vi "Modified Traverse Positions.vi"(4 "Input Position":sgl[](array[numeric])=[0.0, 0.0, 0.0] format="%.2f", 5 "Simulate/Run":T1, 6 "Work in Tunnel Coordinates?":T2, 7 "Extra Command String":string) -> (0 "Error String":string, 1 "XYZ Offset of 2nd Traverse":sgl[](array[numeric]), 2 "Traverse Positions":sgl[][](array[numeric]) format="%.2f", 3 "Traverse Setups":string[](array[string]))   [LabVIEW 2018]
uses:
  Controls/Tunnel_Coordinates.ctl
  Controls/User_Specific_mode.ctl
  Globals/Trav_pos_global.vi
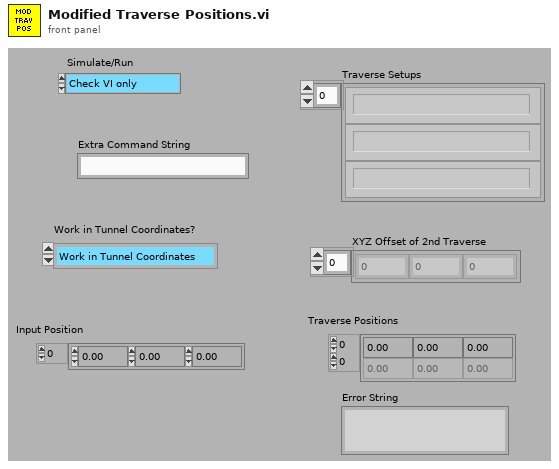
[diagram p1: front panel]
types:
  T1 = typedef "User_Specific_mode.ctl" = enum16{"Check VI only", "Run VI"}
  T2 = typedef "Tunnel_Coordinates.ctl" = enum16{"Work in Tunnel Coordinates", "Work in Model Coordinates"}
  T3 = enum16{"To Traverse Coordinates", "To User Coordinates"}
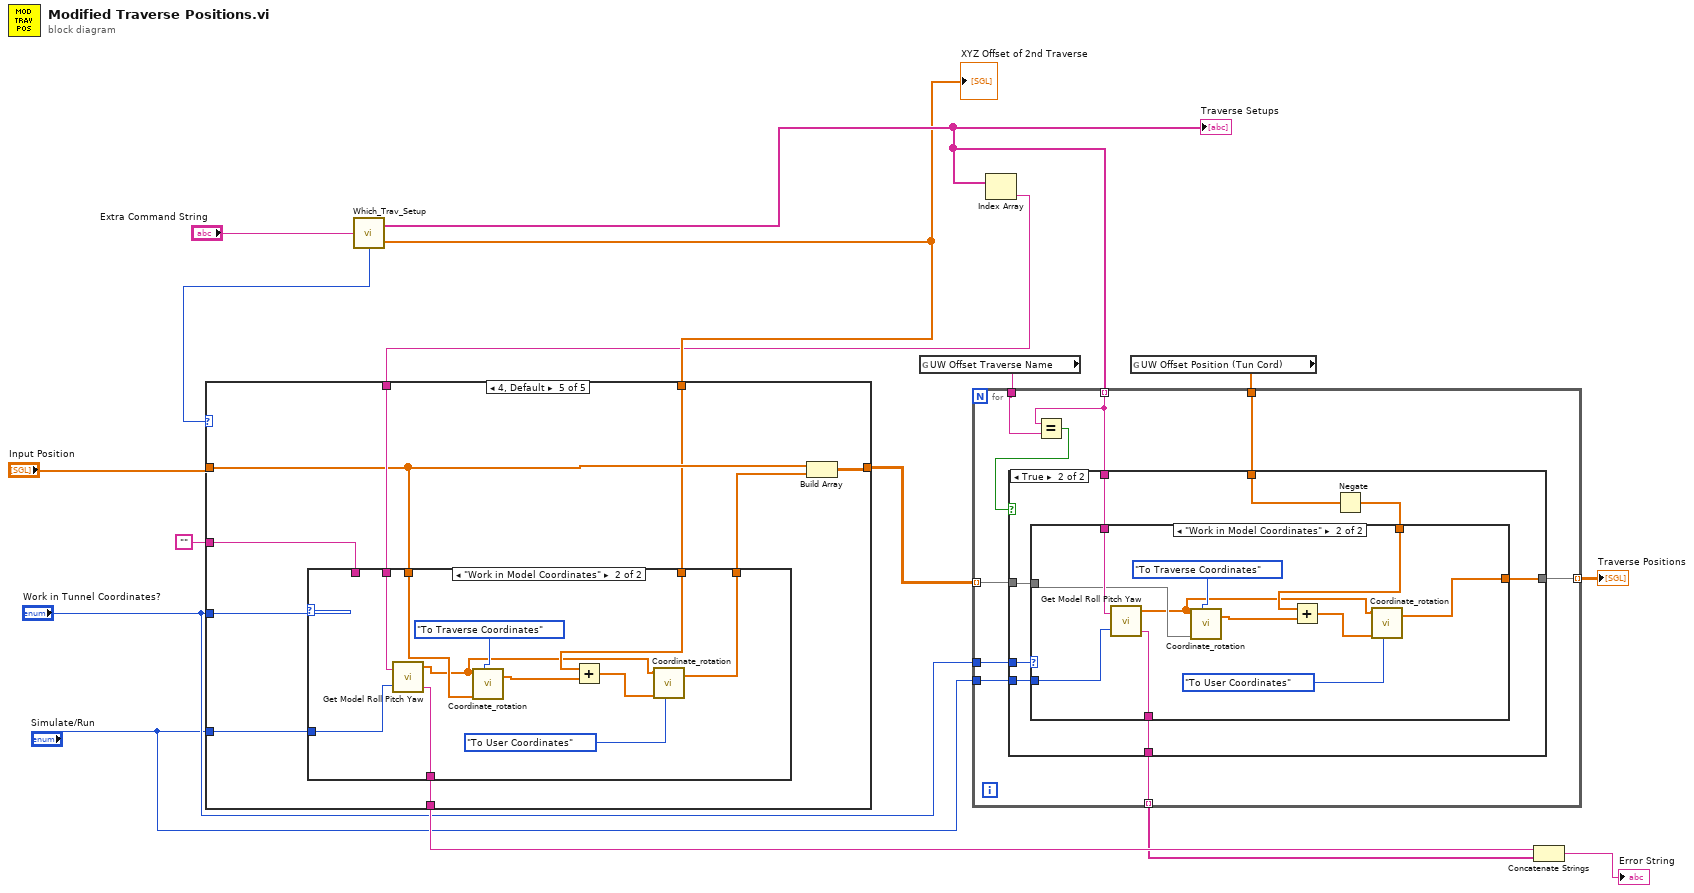
[diagram p0: block diagram]
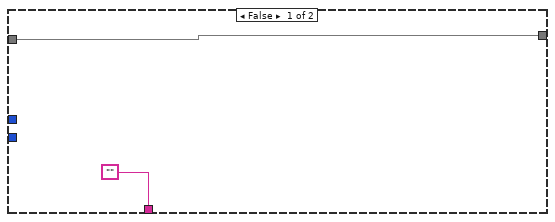
[diagram p2: hidden frame]
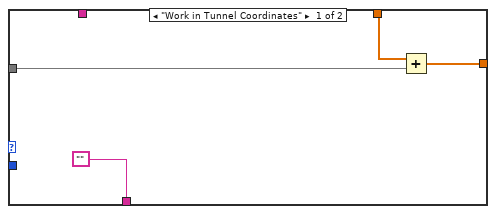
[diagram p3: hidden frame]
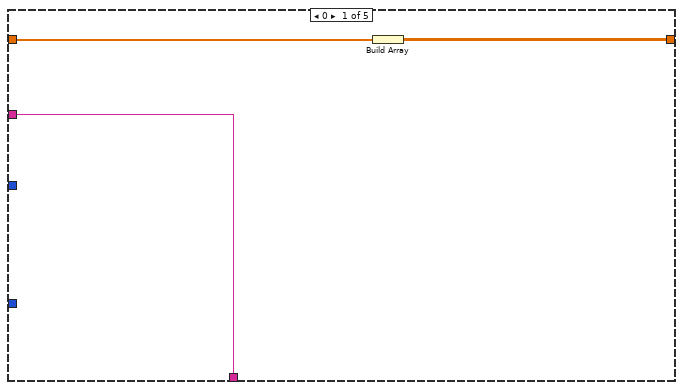
[diagram p4: hidden frame]
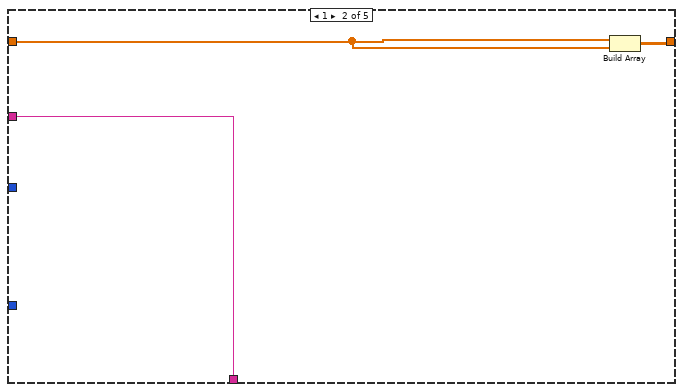
[diagram p5: hidden frame]
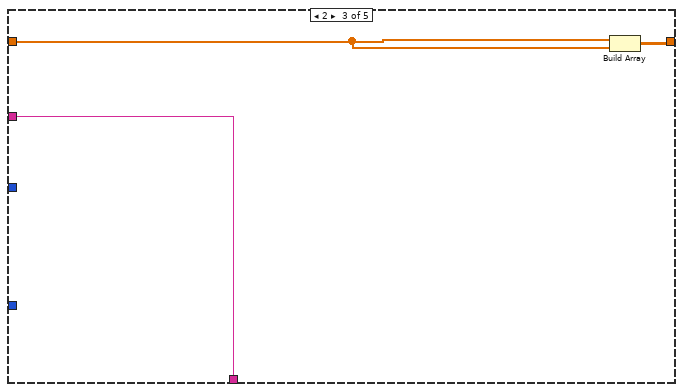
[diagram p6: hidden frame]
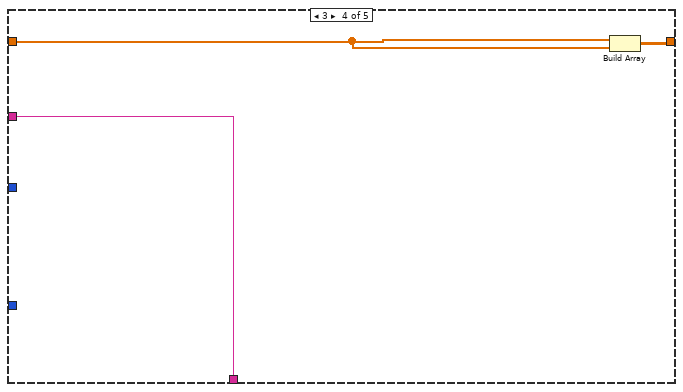
[diagram p7: hidden frame]
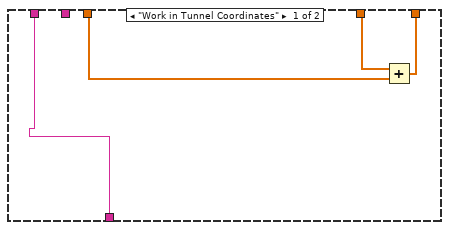
[diagram p8: hidden frame]
diagram:
  n1 = call "Which_Trav_Setup.vi"("Extra Command String"="Extra Command String") -> ("Index"=w12:i32, "Traverse Setups"=w11:string[], "XYZ Offset of 2nd Traverse"=w10:sgl[])
  "Traverse Setups" <- w11
  "XYZ Offset of 2nd Traverse" <- w10
  n2 = global read "Trav_pos_global.vi" "UW Offset Traverse Name"() -> (w1:string)
  n3 = Index Array(array=w11) -> (element=w5:string)  [unwired: 1 in]
  n4 = case shown="4, Default" w12 {
    tunnel: "Input Position" -> [w19 w22 w25 w28 w34]
    tunnel: [w18 w21 w24 w27 w37] -> w15
    tunnel: w10 -> [_ _ _ _ w33]
    tunnel: w5 -> [_ _ _ _ w36]
    tunnel: "Simulate/Run" -> [_ _ _ _ w35]
    tunnel: "Work in Tunnel Coordinates?" -> [_ _ _ _ w31]
    tunnel: [w17 w20 w23 w26 w30] -> w9
    tunnel: "" -> [w17 w20 w23 w26 w29]
    frame 0 {
      n5 = Build Array(w19) -> (w18:sgl[][])
    }
    frame 1 {
      n6 = Build Array(w22, w22) -> (w21:sgl[][])
    }
    frame 2 {
      n7 = Build Array(w25, w25) -> (w24:sgl[][])
    }
    frame 3 {
      n8 = Build Array(w28, w28) -> (w27:sgl[][])
    }
    frame 4, Default {
      n9 = case shown="\"Work in Model Coordinates\"" w31 {
        tunnel: w36 -> [_ w51]
        tunnel: w35 -> [_ w50]
        tunnel: w34 -> [w40 w49]
        tunnel: w33 -> [w41 w47]
        tunnel: [w39 w43] -> w32
        tunnel: [w38 w42] -> w30
        tunnel: w29 -> [w38 _]
        frame "Work in Tunnel Coordinates" {
          n10 = Add(x=w41, y=w40) -> (x+y=w39:sgl[])
        }
        frame "Work in Model Coordinates" {
          n11 = call "Get Model Roll Pitch Yaw.vi"("Traverse Name"=w51, "Mode"=w50) -> ("Model:    Roll        Pitch         Yaw  (deg)"=w46:sgl[], "Error String"=w42:string)  [unwired: 1 out]
          n12 = call "Coordinate_rotation.vi"("Roll-Pitch-Yaw"=w46, "Input Position"=w49, "Mode"=T3."To Traverse Coordinates") -> ("Output Position"=w48:sgl[])  [unwired: 2 in, 1 out]
          n13 = Add(x=w47, y=w48) -> (x+y=w45:sgl[])
          n14 = call "Coordinate_rotation.vi"("Roll-Pitch-Yaw"=w46, "Input Position"=w45, "Mode"=T3."To User Coordinates") -> ("Output Position"=w43:sgl[])  [unwired: 2 in, 1 out]
        }
      }
      n15 = Build Array(w34, w32) -> (w37:sgl[][])
    }
  }
  n16 = global read "Trav_pos_global.vi" "UW Offset Position (Tun Cord)"() -> (w2:sgl[])
  n17 = for {
    tunnel: w11 -> [w59] mode=indexing
    tunnel: "Work in Tunnel Coordinates?" -> [w61]
    tunnel: "Simulate/Run" -> [w60]
    tunnel: w1 -> [w58]
    tunnel: w15 -> [w56] mode=indexing
    tunnel: [w55] -> w14 mode=indexing
    tunnel: [w54] -> w8 mode=indexing
    tunnel: w2 -> [w53]
    n18 = Equal?(x=w59, y=w58) -> (x = y?=w57:bool)
    n19 = case shown="True" w57 {
      tunnel: w59 -> [_ w71]
      tunnel: w61 -> [_ w70]
      tunnel: w60 -> [_ w69]
      tunnel: w56 -> [w63 w68]
      tunnel: [w63 w67] -> w55
      tunnel: ["" w65] -> w54
      tunnel: w53 -> [_ w64]
      frame False {
      }
      frame True {
        n20 = Negate(x=w64) -> (-x=w66:sgl[])
        n21 = case shown="\"Work in Model Coordinates\"" w70 {
          tunnel: w71 -> [_ w85]
          tunnel: w69 -> [_ w84]
          tunnel: w68 -> [w74 w83]
          tunnel: w66 -> [w75 w81]
          tunnel: [w73 w77] -> w67
          tunnel: ["" w76] -> w65
          frame "Work in Tunnel Coordinates" {
            n22 = Add(x=w75, y=w74) -> (x+y=w73:sgl[])
          }
          frame "Work in Model Coordinates" {
            n23 = call "Get Model Roll Pitch Yaw.vi"("Traverse Name"=w85, "Mode"=w84) -> ("Model:    Roll        Pitch         Yaw  (deg)"=w80:sgl[], "Error String"=w76:string)  [unwired: 1 out]
            n24 = call "Coordinate_rotation.vi"("Roll-Pitch-Yaw"=w80, "Input Position"=w83, "Mode"=T3."To Traverse Coordinates") -> ("Output Position"=w82:sgl[])  [unwired: 2 in, 1 out]
            n25 = Add(x=w81, y=w82) -> (x+y=w79:sgl[])
            n26 = call "Coordinate_rotation.vi"("Roll-Pitch-Yaw"=w80, "Input Position"=w79, "Mode"=T3."To User Coordinates") -> ("Output Position"=w77:sgl[])  [unwired: 2 in, 1 out]
          }
        }
      }
    }
  }
  "Traverse Positions" <- w14
  n27 = Concatenate Strings(w9, w8) -> (→"Error String":string)
